vi "Test Customer Order Sent to Handler on Submit Order.vi"(8 "error in (no error)":errorcluster, 11 "Customer Test in":refnum<class "Customer Test.lvclass">) -> (0 "error out":errorcluster, 3 "Customer Test out":refnum<class "Customer Test.lvclass">)   [LabVIEW 2020, in "Customer Test.lvclass"]
uses:
  Customer Test.lvclass
  C:/Program Files (x86)/National Instruments/LabVIEW 2020/vi.lib/Asteme/LUnit/Test Case.lvclass
  Processes/People/Customers/Customer/Customer.lvclass
  C:/Program Files (x86)/National Instruments/LabVIEW 2020/vi.lib/Asteme/Triarc Framework/Process/Process.lvclass
  Support/Beverages/TypeDefs/Drink Type.ctl
  Support/Beverages/TypeDefs/Options.ctl
  Test Doubles/Mock Job Handler/Mock Job Handler.lvclass
  C:/Users/anton/Documents/GitHub/Triarc-Examples/Coffee Shop/Process Job/Job Handler.lvclass
  <vilib>/Asteme/Triarc Framework/Process/Process.lvclass/Process.ctl
  <vilib>/Asteme/LUnit/Test Case.lvclass/Test Case.ctl
  <vilib>/Asteme/LUnit/LUnit Assertion Result.lvclass/LUnit Assertion Result.ctl
  <vilib>/Asteme/Triarc Framework/Process/Private/SubVIs/Wait for finish.vi
  <vilib>/Asteme/Triarc Framework/Process/Protected/Messaging/Enqueue Message.vi
  <vilib>/Asteme/Triarc Framework/Process/Private/SubVIs/Set Lifecycle State.vi
  <vilib>/Asteme/Triarc Framework/Process/Public/Lifecycle/Get Lifecycle State.vi
  <vilib>/Asteme/LUnit/Palette/Pass If.vi
  <vilib>/Asteme/LUnit/Set Assertion Type.vi
  <vilib>/AdvancedString/1D String Array to Delimited String.vi
  <vilib>/Utility/error.llb/Clear Errors.vi
  <vilib>/Asteme/LUnit/Palette/Fail.vi
  <vilib>/Asteme/LUnit/Palette/Pass.vi
  <vilib>/Asteme/LUnit/LUnit Write Assertion Type.vi
  <vilib>/Asteme/LUnit/Add test result.vi
  <vilib>/Asteme/LUnit/LUnit Write Passed.vi
  <vilib>/Asteme/LUnit/LUnit Get Test Case.vi
  <vilib>/Asteme/LUnit/Assertion Result/LUnit Get Test Name.vi
  <vilib>/Asteme/LUnit/LUnit Write Message.vi
  <vilib>/Asteme/LUnit/LUnit Write Description.vi
  <vilib>/Asteme/LUnit/Read Test Case Name.vi
  <vilib>/Utility/error.llb/Error Cluster From Error Code.vi
  <vilib>/Asteme/LUnit/LUnit Assertion Result.lvclass
  <vilib>/Asteme/Triarc Framework/Process/Process.lvclass
  Support/Beverages/Beverage/Beverage.lvclass
  <vilib>/Asteme/LUnit/Test Case.lvclass
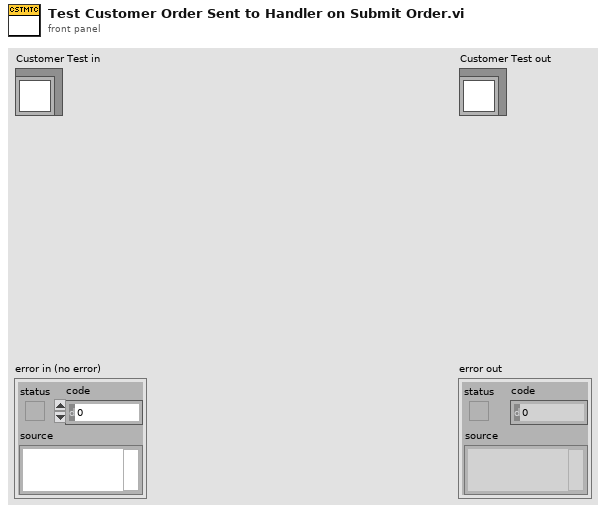
[diagram p1: front panel]
types:
  T1 = typedef "Beverage.lvclass/Drink Type.ctl" = enum16{"Dark Roast", "Decaf", "Espresso", "House Blend"}
  T2 = typedef "Beverage.lvclass/Options.ctl" = enum16{"<None>", "Milk", "Mocha", "Soy", "Whip"}
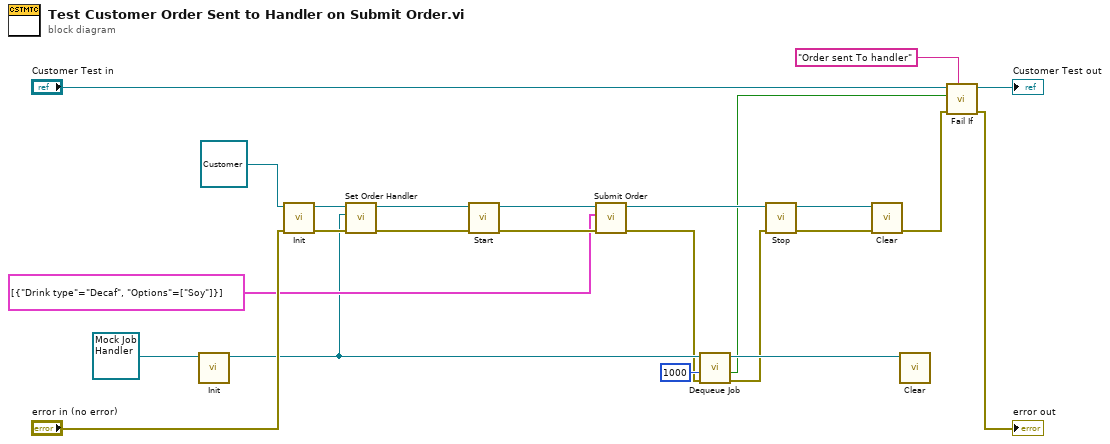
[diagram p0: block diagram]
diagram:
  n1 = call-dynamic "Init.vi"("Mock Job Handler In"=refnum<class "Mock Job Handler.lvclass"> refnum ("Mock Job Handler.lvclass")) -> ("Mock Job Handler Out"=w5:refnum<class "Mock Job Handler.lvclass">)  [unwired: 9 in, 1 out]
  n2 = call-dynamic "Init.vi"("error in (no error)"="error in (no error)", "View In"=refnum<class "Customer.lvclass"> refnum ("Customer.lvclass")) -> ("error out"=w23:errorcluster, "View Out"=w9:refnum<class "Customer.lvclass">)  [unwired: 8 in]
  n3 = call "Set Order Handler.vi"("error in (no error)"=w23, "Order Handler"=w5, "Customer In"=w9) -> ("error out"=w10:errorcluster, "Customer Out"=w8:refnum<class "Customer.lvclass">)  [unwired: 7 in]
  n4 = call <vilib>:"Start.vi"("error in (no error)"=w10, "Process In"=w8) -> ("error out"=w17:errorcluster, "Process Out"=w19:refnum<class "Customer.lvclass">)  [unwired: 8 in]
  n5 = call "Submit Order.vi"("error in (no error)"=w17, "Order Content"=cluster{"Drink type":T1, "Options":T2[]}[] [{"Drink type"=enum."Decaf", "Options"=[enum."Soy"]}] ("Order"), "Customer In"=w19) -> ("error out"=w2:errorcluster, "Customer Out"=w18:refnum<class "Customer.lvclass">)  [unwired: 7 in]
  n6 = call "Dequeue Job.vi"("error in (no error)"=w2, "timeout in ms (-1)"=1000, "Mock Job Handler In"=w5) -> ("error out"=w1:errorcluster, "timed out?"=w3:bool, "Mock Job Handler Out"=w7:refnum<class "Mock Job Handler.lvclass">)  [unwired: 5 in, 1 out]
  n7 = call <vilib>:"Stop.vi"("error in (no error)"=w1, "Process In"=w18) -> ("error out"=w21:errorcluster, "Process Out"=w22:refnum<class "Customer.lvclass">)  [unwired: 7 in, 1 out]
  n8 = call-dynamic "Clear.vi"("error in (no error)"=w21, "View In"=w22) -> ("error out"=w14:errorcluster)  [unwired: 9 in]
  n9 = call-dynamic "Clear.vi"("Mock Job Handler In"=w7) -> ()  [unwired: 10 in, 1 out]
  n10 = call <vilib>:"Fail If.vi"("Description"="Order sent To handler", "error in (no error)"=w14, "Fail?"=w3, "Test Case In"="Customer Test in") -> ("error out"=→"error out":errorcluster, "Test Case Out"=→"Customer Test out":refnum<class "Customer Test.lvclass">)  [unwired: 6 in]
